vi "encodeUInt32.vi"(2 "Compress? (T)":bool=TRUE, 3 "UInt32":u32) -> (1 "MessagePack":u8[](array[numeric]) format="%.0x")   [LabVIEW 2015, in "MsgPack.lvlib"]
uses:
  MsgPack.lvlib
  encodeUInt8.vi
  SubVis/encodeFixedInt.vi
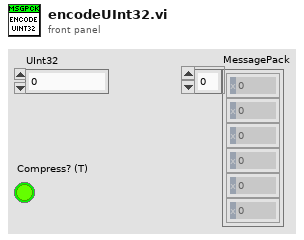
[diagram p1: front panel]
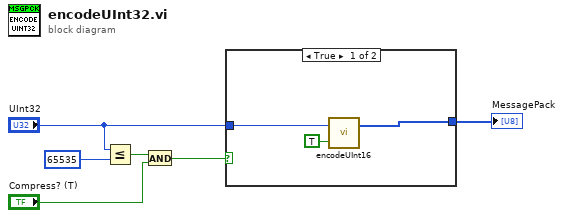
[diagram p0: block diagram]
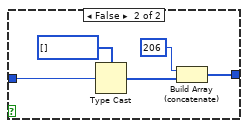
[diagram p2: hidden frame]
diagram:
  n1 = Less Or Equal?(x="UInt32", y=u32 65535) -> (x <= y?=w4:bool)
  n2 = And(x=w4, y="Compress? (T)") -> (x .and. y?=w1:bool)
  n3 = case shown="True" w1 {
    tunnel: [w9 w14] -> w6
    tunnel: "UInt32" -> [w8 w10]
    frame True {
      n4 = call "encodeUInt16.vi"("Compress? (T)"=TRUE ("Compress"), "UInt16"=w8) -> ("MessagePack"=w9:u8[])  [unwired: 1 in]
    }
    frame False {
      n5 = Type Cast(type=u8[] [], x=w10) -> (*(type *) &x=w11:u8[])
      n6 = Build Array (concatenate)(u8 206, w11) -> (w14:u8[])
    }
  }
  "MessagePack" <- w6
